vi "SBML Events Handler.vi"(0 "Sim Data w/ time":dbl[][](array[numeric]), 1 "Math Op":string[](array[string]), 2 "Math Val":string[](array[string]), 3 "Var Idx":i32[](array[numeric]), 4 "Idx of Time":i32, 5 "Assign Val":string[][](array[string]), 6 "Delay":dbl[](array[numeric]), 7 "Assign Var Idx":i32[][](array[numeric]), 8 "Flag":i32[](array[numeric]), 9 "Priority":dbl[](array[numeric]), 10 "Delay Val Tot":dbl[](array[numeric]), 11 "Delay Val":dbl) -> (16 "Output Data":dbl[][](array[numeric]), 18 "Flag Out":i32[](array[numeric]), 19 "Delay Val Tot Out":dbl[](array[numeric]))   [LabVIEW 2014]
uses:
  Stop ODE.vi
panel:
  out "Event Idx":i32
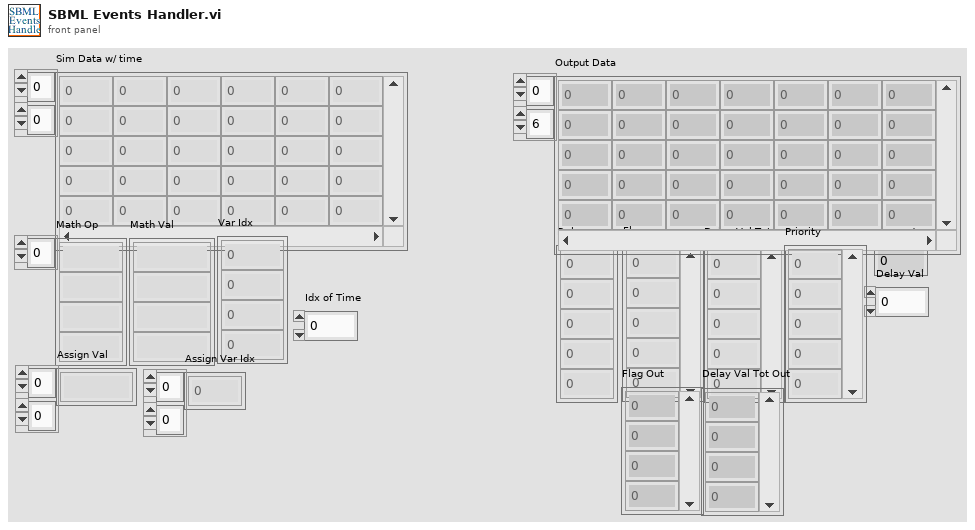
[diagram p1: front panel]
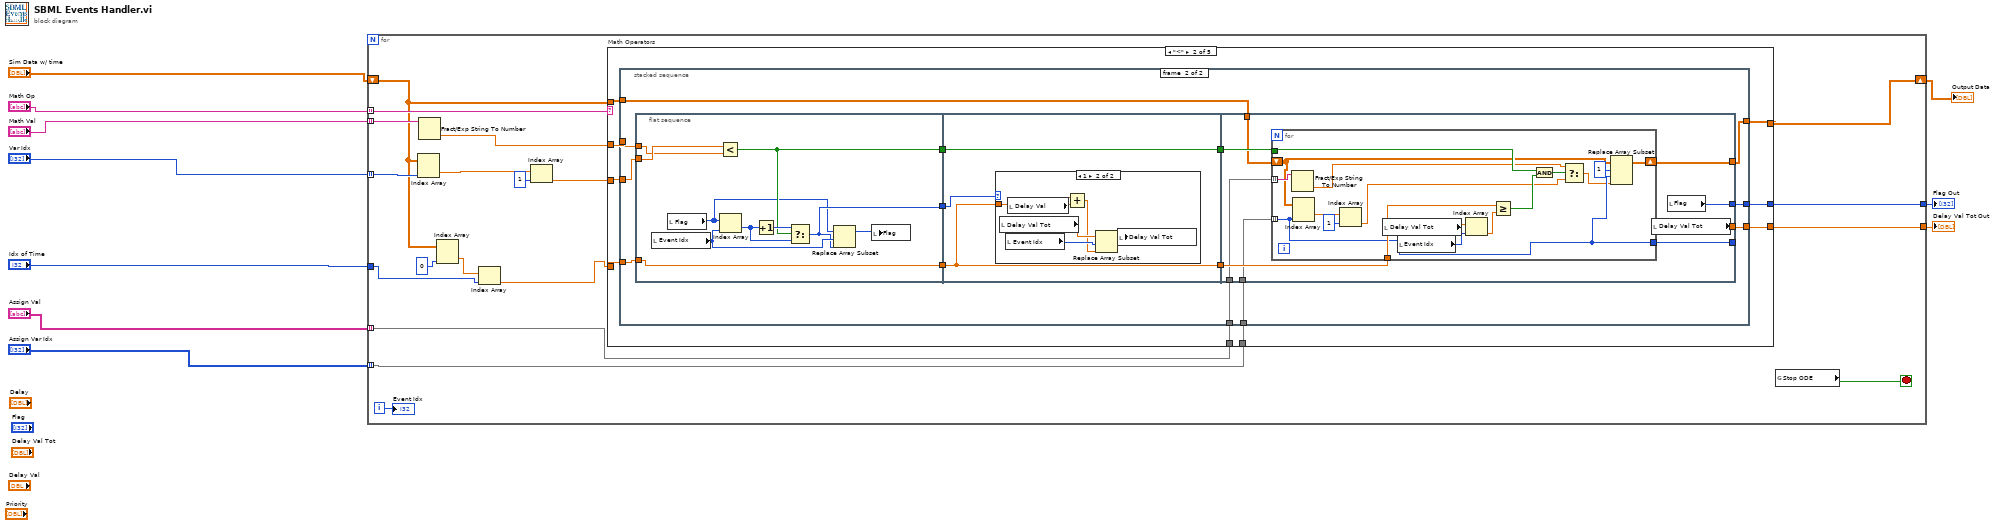
[diagram p0: block diagram]
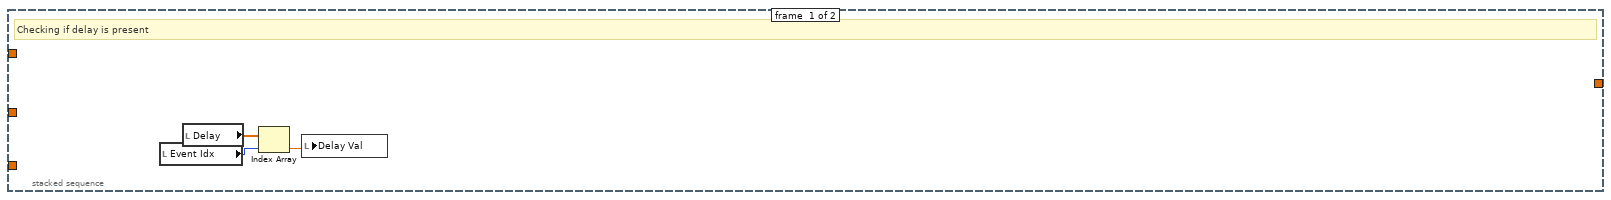
[diagram p3: hidden frame]
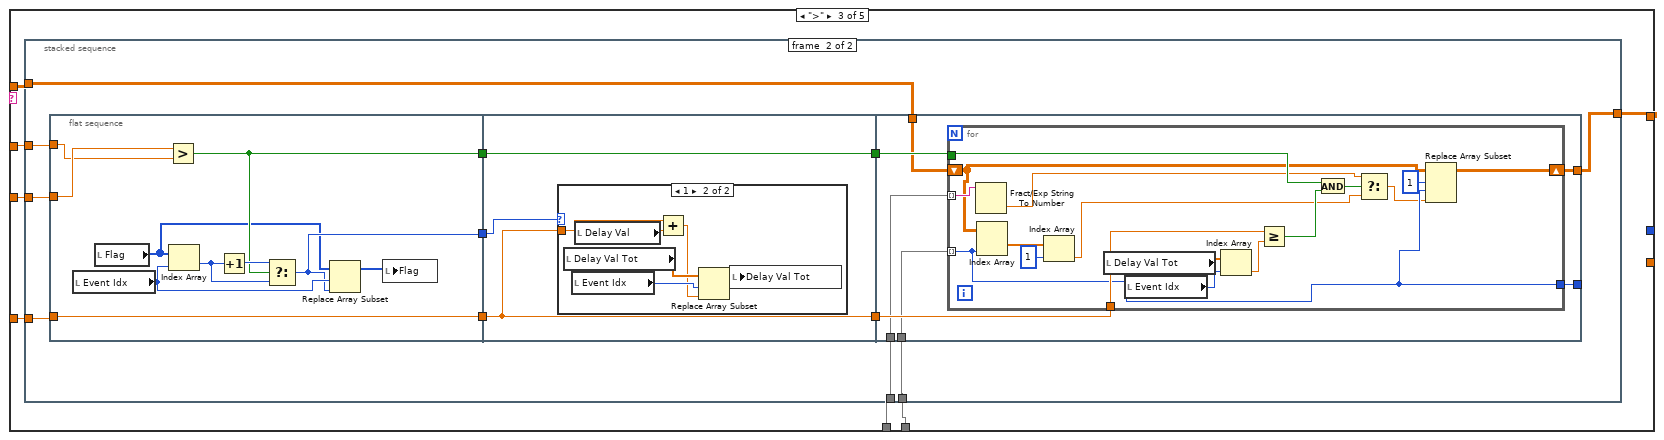
[diagram p5: hidden frame]
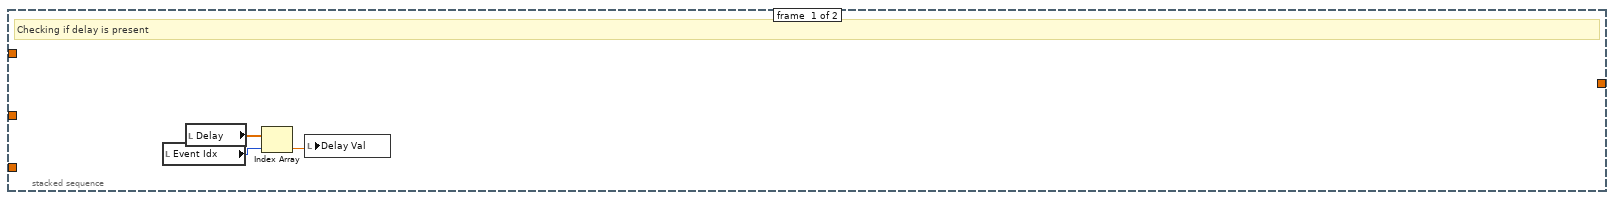
[diagram p6: hidden frame]
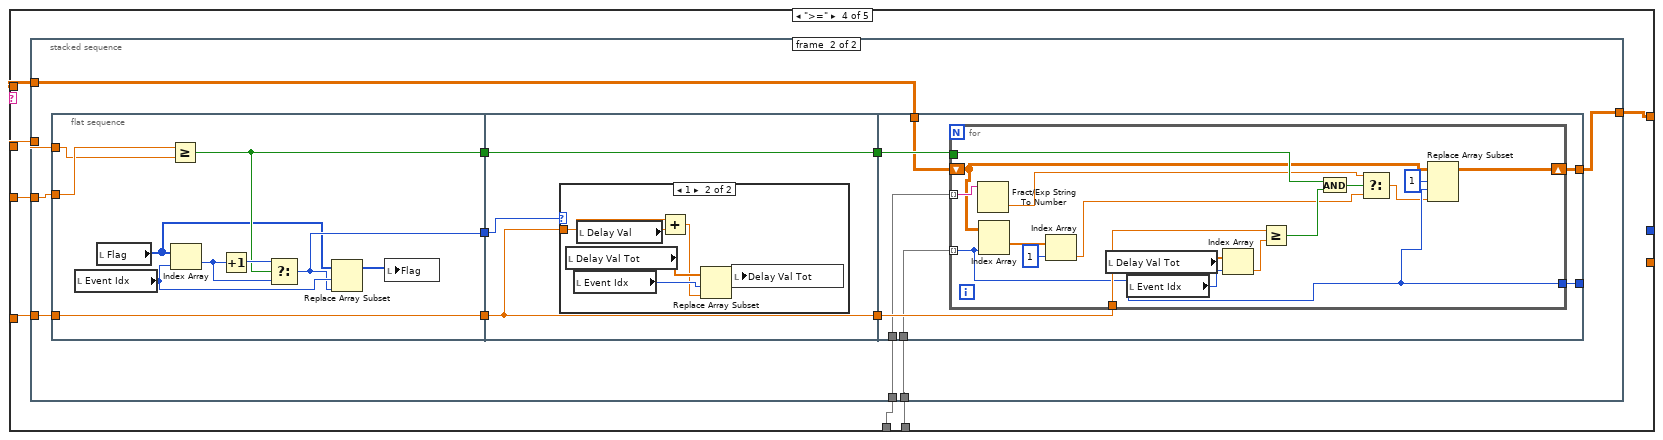
[diagram p8: hidden frame]
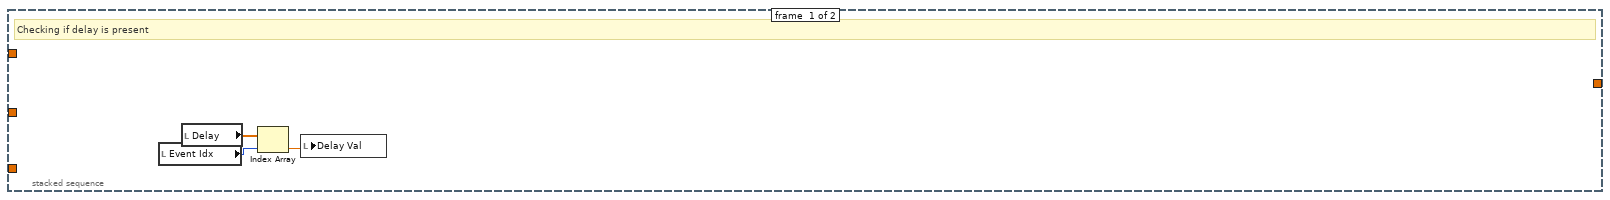
[diagram p9: hidden frame]
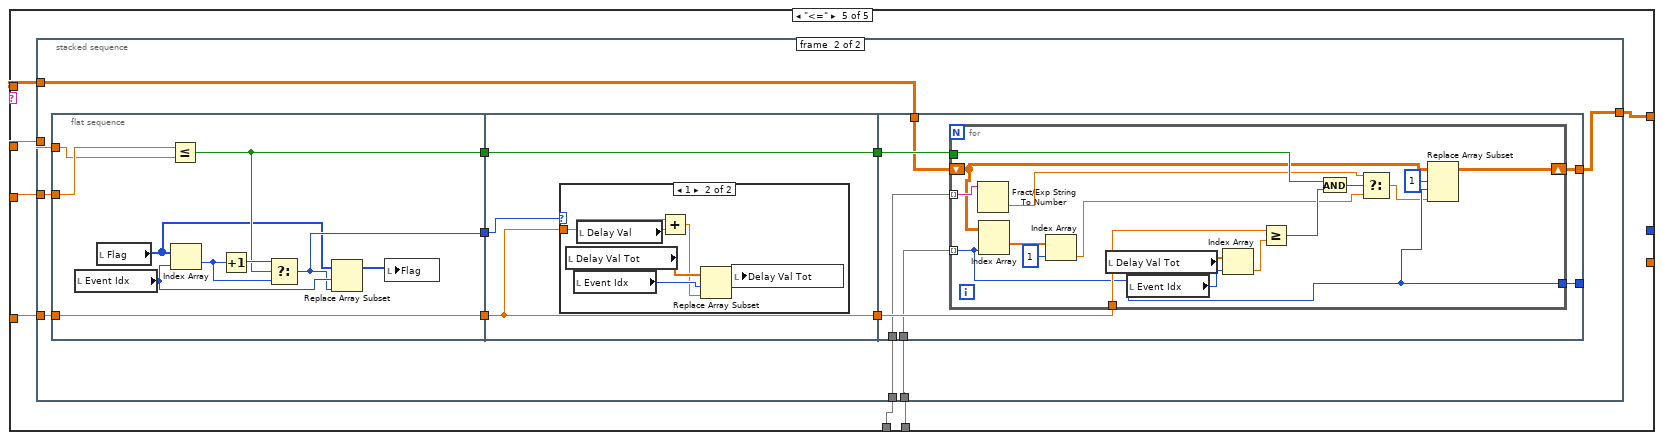
[diagram p11: hidden frame]
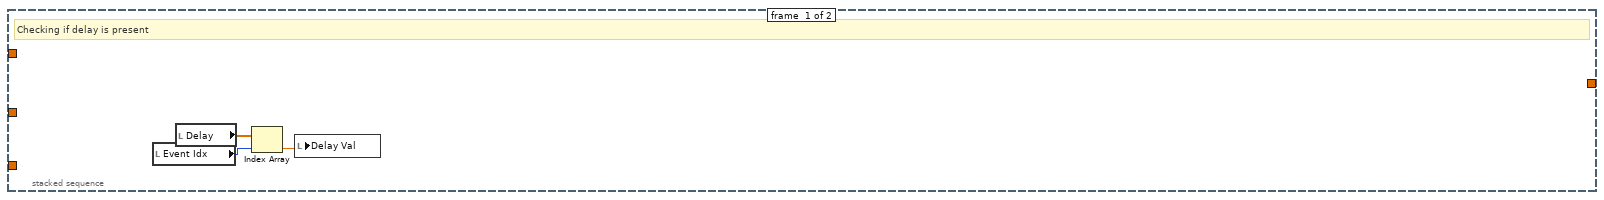
[diagram p12: hidden frame]
diagram:
  n1 = for {
    tunnel: "Math Op" -> [w29] mode=indexing
    tunnel: "Math Val" -> [w28] mode=indexing
    tunnel: "Var Idx" -> [w27] mode=indexing
    tunnel: "Assign Val" -> [w23] mode=indexing
    tunnel: "Assign Var Idx" -> [w26] mode=indexing
    shift-right: [w21] -> w10
    shift-left: "Sim Data w/ time" -> [w15]
    tunnel: "Idx of Time" -> [w13]
    tunnel: [w12] -> w2
    tunnel: [w11] -> w1
    i -> [w24]
    stop <- w25 stop-if-true
    n2 = Index Array(array=w15, index (col)=w27) -> (element=w19:dbl[])  [unwired: 1 in]
    n3 = Fract/Exp String To Number(string=w28) -> (number=w22:dbl)  [unwired: 3 in, 1 out]
    n4 = Index Array(array=w15, index (col)=0 ("disabled index (col)")) -> (element=w17:dbl[])  [unwired: 1 in]
    n5 = Index Array(array=w17, index=w13) -> (element=w14:dbl)
    n6 = Index Array(array=w19, index=1) -> (element=w18:dbl)
    n7 = case "Math Operators" shown="\"<\"" w29 {
      tunnel: w22 -> [_ w37 w106 w171 w236]
      tunnel: [_ w36 w105 w170 w235] -> w21
      tunnel: w15 -> [_ w38 w107 w172 w237]
      tunnel: w23 -> [_ w35 w104 w169 w234]
      tunnel: w26 -> [_ w34 w103 w168 w233]
      tunnel: w18 -> [_ w33 w102 w166 w232]
      tunnel: w14 -> [_ w32 w101 w167 w231]
      tunnel: [_ w31 _ _ _] -> w12
      tunnel: [_ w30 _ _ _] -> w11
      frame "False", Default {
      }
      frame "<" {
        n8 = stacked-sequence {
          tunnel: w37 -> [_ w55]
          tunnel: w38 -> [_ w47]
          tunnel: [_ w46] -> w36
          tunnel: w35 -> [_ w49]
          tunnel: w34 -> [_ w48]
          tunnel: w33 -> [_ w45]
          tunnel: w32 -> [_ w44]
          tunnel: [_ w43] -> w31
          tunnel: [_ w42] -> w30
          frame #0 {
            # "Checking if delay is present"
            n9 = local read "Event Idx"() -> (w40:i32)
            n10 = local read "Delay"() -> (w41:dbl[])
            n11 = Index Array(array=w41, index=w40) -> (element=w39:dbl)
            n12 = local write "Delay Val"(w39) -> ()
          }
          frame #1 {
            n13 = flat-sequence {
              tunnel: w45 -> [w65]
              tunnel: w55 -> [w64]
              tunnel: [w59] -> w54
              tunnel: [w58] -> w53
              tunnel: [w56] -> w52
              tunnel: w44 -> [w56]
              tunnel: w54 -> [w67]
              tunnel: w53 -> [w68]
              tunnel: w52 -> [w66]
              tunnel: [w68] -> w51
              tunnel: [w66] -> w50
              tunnel: w51 -> [w83]
              tunnel: w50 -> [w82]
              tunnel: w47 -> [w81]
              tunnel: w48 -> [w80]
              tunnel: w49 -> [w79]
              tunnel: [w78] -> _
              tunnel: [w77] -> w46
              tunnel: [w76] -> w43
              tunnel: [w75] -> w42
              frame #0 {
                n14 = local read "Event Idx"() -> (w62:i32)
                n15 = local read "Flag"() -> (w57:i32[])
                n16 = Less?(x=w65, y=w64) -> (x < y?=w58:bool)
                n17 = Index Array(array=w57, index=w62) -> (element=w61:i32)
                n18 = Increment(x=w61) -> (x+1=w60:i32)
                n19 = Select(t=w60, s=w58, f=w61) -> (s? t:f=w59:i32)
                n20 = Replace Array Subset(array=w57, new element=w59, index=w62) -> (w63:i32[])
                n21 = local write "Flag"(w63) -> ()
              }
              frame #1 {
                n22 = case shown="1" w67 {
                  tunnel: w66 -> [_ w73]
                  frame 0, Default {
                  }
                  frame 1 {
                    n23 = local read "Delay Val Tot"() -> (w72:dbl[])
                    n24 = local read "Event Idx"() -> (w70:i32)
                    n25 = local read "Delay Val"() -> (w74:dbl)
                    n26 = Add(x=w73, y=w74) -> (x+y=w69:dbl)
                    n27 = Replace Array Subset(array=w72, new element=w69, index=w70) -> (w71:dbl[])
                    n28 = local write "Delay Val Tot"(w71) -> ()
                  }
                }
              }
              frame #2 {
                n29 = for {
                  tunnel: w83 -> [w98]
                  tunnel: w82 -> [w97]
                  tunnel: w80 -> [w87] mode=indexing
                  tunnel: w79 -> [w90] mode=indexing
                  tunnel: [w87] -> w78
                  shift-right: [w85] -> w77
                  shift-left: w81 -> [w84]
                  n30 = Fract/Exp String To Number(string=w90) -> (number=w89:dbl)  [unwired: 3 in, 1 out]
                  n31 = Index Array(array=w84, index (col)=w87) -> (element=w92:dbl[])  [unwired: 1 in]
                  n32 = Index Array(array=w92, index=1) -> (element=w91:dbl)
                  n33 = local read "Delay Val Tot"() -> (w96:dbl[])
                  n34 = local read "Event Idx"() -> (w95:i32)
                  n35 = Index Array(array=w96, index=w95) -> (element=w94:dbl)
                  n36 = Greater Or Equal?(x=w97, y=w94) -> (x >= y?=w99:bool)
                  n37 = And(x=w98, y=w99) -> (x .and. y?=w100:bool)
                  n38 = Select(t=w89, s=w100, f=w91) -> (s? t:f=w86:dbl)
                  n39 = Replace Array Subset(array=w84, new element=w86, index (row)=1, index (col)=w87) -> (w85:dbl[][])
                }
                n40 = local read "Delay Val Tot"() -> (w75:dbl[])
                n41 = local read "Flag"() -> (w76:i32[])
              }
            }
          }
        }
      }
      frame ">" {
        n42 = stacked-sequence {
          tunnel: w106 -> [_ w122]
          tunnel: w107 -> [_ w114]
          tunnel: [_ w113] -> w105
          tunnel: w104 -> [_ w116]
          tunnel: w103 -> [_ w115]
          tunnel: w102 -> [_ w112]
          tunnel: w101 -> [_ w111]
          frame #0 {
            # "Checking if delay is present"
            n43 = local read "Event Idx"() -> (w109:i32)
            n44 = local read "Delay"() -> (w110:dbl[])
            n45 = Index Array(array=w110, index=w109) -> (element=w108:dbl)
            n46 = local write "Delay Val"(w108) -> ()
          }
          frame #1 {
            n47 = flat-sequence {
              tunnel: w112 -> [w132]
              tunnel: w122 -> [w131]
              tunnel: w111 -> [w130]
              tunnel: [w125] -> w121
              tunnel: [w124] -> w120
              tunnel: [w130] -> w119
              tunnel: w121 -> [w134]
              tunnel: w120 -> [w135]
              tunnel: w119 -> [w133]
              tunnel: [w135] -> w118
              tunnel: [w133] -> w117
              tunnel: w118 -> [w148]
              tunnel: w117 -> [w147]
              tunnel: w114 -> [w146]
              tunnel: w115 -> [w145]
              tunnel: w116 -> [w144]
              tunnel: [w143] -> _
              tunnel: [w142] -> w113
              frame #0 {
                n48 = local read "Event Idx"() -> (w128:i32)
                n49 = local read "Flag"() -> (w123:i32[])
                n50 = Greater?(x=w132, y=w131) -> (0:w124:bool)
                n51 = Index Array(array=w123, index=w128) -> (element=w127:i32)
                n52 = Increment(x=w127) -> (x+1=w126:i32)
                n53 = Select(t=w126, s=w124, f=w127) -> (s? t:f=w125:i32)
                n54 = Replace Array Subset(array=w123, new element=w125, index=w128) -> (w129:i32[])
                n55 = local write "Flag"(w129) -> ()
              }
              frame #1 {
                n56 = case shown="1" w134 {
                  tunnel: w133 -> [_ w140]
                  frame 0, Default {
                  }
                  frame 1 {
                    n57 = local read "Delay Val Tot"() -> (w139:dbl[])
                    n58 = local read "Event Idx"() -> (w137:i32)
                    n59 = local read "Delay Val"() -> (w141:dbl)
                    n60 = Add(x=w140, y=w141) -> (x+y=w136:dbl)
                    n61 = Replace Array Subset(array=w139, new element=w136, index=w137) -> (w138:dbl[])
                    n62 = local write "Delay Val Tot"(w138) -> ()
                  }
                }
              }
              frame #2 {
                n63 = for {
                  tunnel: w148 -> [w163]
                  tunnel: w147 -> [w162]
                  tunnel: w145 -> [w152] mode=indexing
                  tunnel: w144 -> [w155] mode=indexing
                  tunnel: [w152] -> w143
                  shift-right: [w150] -> w142
                  shift-left: w146 -> [w149]
                  n64 = Fract/Exp String To Number(string=w155) -> (number=w154:dbl)  [unwired: 3 in, 1 out]
                  n65 = Index Array(array=w149, index (col)=w152) -> (element=w157:dbl[])  [unwired: 1 in]
                  n66 = Index Array(array=w157, index=1) -> (element=w156:dbl)
                  n67 = local read "Delay Val Tot"() -> (w161:dbl[])
                  n68 = local read "Event Idx"() -> (w160:i32)
                  n69 = Index Array(array=w161, index=w160) -> (element=w159:dbl)
                  n70 = Greater Or Equal?(x=w162, y=w159) -> (x >= y?=w164:bool)
                  n71 = And(x=w163, y=w164) -> (x .and. y?=w165:bool)
                  n72 = Select(t=w154, s=w165, f=w156) -> (s? t:f=w151:dbl)
                  n73 = Replace Array Subset(array=w149, new element=w151, index (row)=1, index (col)=w152) -> (w150:dbl[][])
                }
              }
            }
          }
        }
      }
      frame ">=" {
        n74 = stacked-sequence {
          tunnel: w171 -> [_ w187]
          tunnel: w172 -> [_ w179]
          tunnel: [_ w178] -> w170
          tunnel: w169 -> [_ w181]
          tunnel: w168 -> [_ w180]
          tunnel: w167 -> [_ w177]
          tunnel: w166 -> [_ w176]
          frame #0 {
            # "Checking if delay is present"
            n75 = local read "Event Idx"() -> (w174:i32)
            n76 = local read "Delay"() -> (w175:dbl[])
            n77 = Index Array(array=w175, index=w174) -> (element=w173:dbl)
            n78 = local write "Delay Val"(w173) -> ()
          }
          frame #1 {
            n79 = flat-sequence {
              tunnel: w176 -> [w197]
              tunnel: w187 -> [w196]
              tunnel: w177 -> [w195]
              tunnel: [w190] -> w186
              tunnel: [w189] -> w185
              tunnel: [w195] -> w184
              tunnel: w186 -> [w199]
              tunnel: w185 -> [w200]
              tunnel: w184 -> [w198]
              tunnel: [w200] -> w183
              tunnel: [w198] -> w182
              tunnel: w183 -> [w213]
              tunnel: w182 -> [w212]
              tunnel: w179 -> [w211]
              tunnel: w180 -> [w210]
              tunnel: w181 -> [w209]
              tunnel: [w208] -> _
              tunnel: [w207] -> w178
              frame #0 {
                n80 = local read "Event Idx"() -> (w193:i32)
                n81 = local read "Flag"() -> (w188:i32[])
                n82 = Greater Or Equal?(x=w197, y=w196) -> (x >= y?=w189:bool)
                n83 = Index Array(array=w188, index=w193) -> (element=w192:i32)
                n84 = Increment(x=w192) -> (x+1=w191:i32)
                n85 = Select(t=w191, s=w189, f=w192) -> (s? t:f=w190:i32)
                n86 = Replace Array Subset(array=w188, new element=w190, index=w193) -> (w194:i32[])
                n87 = local write "Flag"(w194) -> ()
              }
              frame #1 {
                n88 = case shown="1" w199 {
                  tunnel: w198 -> [_ w205]
                  frame 0, Default {
                  }
                  frame 1 {
                    n89 = local read "Delay Val Tot"() -> (w204:dbl[])
                    n90 = local read "Event Idx"() -> (w202:i32)
                    n91 = local read "Delay Val"() -> (w206:dbl)
                    n92 = Add(x=w205, y=w206) -> (x+y=w201:dbl)
                    n93 = Replace Array Subset(array=w204, new element=w201, index=w202) -> (w203:dbl[])
                    n94 = local write "Delay Val Tot"(w203) -> ()
                  }
                }
              }
              frame #2 {
                n95 = for {
                  tunnel: w213 -> [w228]
                  tunnel: w212 -> [w227]
                  tunnel: w210 -> [w217] mode=indexing
                  tunnel: w209 -> [w220] mode=indexing
                  tunnel: [w217] -> w208
                  shift-right: [w215] -> w207
                  shift-left: w211 -> [w214]
                  n96 = Fract/Exp String To Number(string=w220) -> (number=w219:dbl)  [unwired: 3 in, 1 out]
                  n97 = Index Array(array=w214, index (col)=w217) -> (element=w222:dbl[])  [unwired: 1 in]
                  n98 = Index Array(array=w222, index=1) -> (element=w221:dbl)
                  n99 = local read "Delay Val Tot"() -> (w226:dbl[])
                  n100 = local read "Event Idx"() -> (w225:i32)
                  n101 = Index Array(array=w226, index=w225) -> (element=w224:dbl)
                  n102 = Greater Or Equal?(x=w227, y=w224) -> (x >= y?=w229:bool)
                  n103 = And(x=w228, y=w229) -> (x .and. y?=w230:bool)
                  n104 = Select(t=w219, s=w230, f=w221) -> (s? t:f=w216:dbl)
                  n105 = Replace Array Subset(array=w214, new element=w216, index (row)=1, index (col)=w217) -> (w215:dbl[][])
                }
              }
            }
          }
        }
      }
      frame "<=" {
        n106 = stacked-sequence {
          tunnel: w236 -> [_ w252]
          tunnel: w237 -> [_ w244]
          tunnel: [_ w243] -> w235
          tunnel: w234 -> [_ w246]
          tunnel: w233 -> [_ w245]
          tunnel: w232 -> [_ w242]
          tunnel: w231 -> [_ w241]
          frame #0 {
            # "Checking if delay is present"
            n107 = local read "Event Idx"() -> (w239:i32)
            n108 = local read "Delay"() -> (w240:dbl[])
            n109 = Index Array(array=w240, index=w239) -> (element=w238:dbl)
            n110 = local write "Delay Val"(w238) -> ()
          }
          frame #1 {
            n111 = flat-sequence {
              tunnel: w242 -> [w262]
              tunnel: w252 -> [w261]
              tunnel: w241 -> [w260]
              tunnel: [w255] -> w251
              tunnel: [w254] -> w250
              tunnel: [w260] -> w249
              tunnel: w251 -> [w264]
              tunnel: w250 -> [w265]
              tunnel: w249 -> [w263]
              tunnel: [w265] -> w248
              tunnel: [w263] -> w247
              tunnel: w248 -> [w278]
              tunnel: w247 -> [w277]
              tunnel: w244 -> [w276]
              tunnel: w245 -> [w275]
              tunnel: w246 -> [w274]
              tunnel: [w273] -> _
              tunnel: [w272] -> w243
              frame #0 {
                n112 = local read "Event Idx"() -> (w258:i32)
                n113 = local read "Flag"() -> (w253:i32[])
                n114 = Less Or Equal?(x=w262, y=w261) -> (x <= y?=w254:bool)
                n115 = Index Array(array=w253, index=w258) -> (element=w257:i32)
                n116 = Increment(x=w257) -> (x+1=w256:i32)
                n117 = Select(t=w256, s=w254, f=w257) -> (s? t:f=w255:i32)
                n118 = Replace Array Subset(array=w253, new element=w255, index=w258) -> (w259:i32[])
                n119 = local write "Flag"(w259) -> ()
              }
              frame #1 {
                n120 = case shown="1" w264 {
                  tunnel: w263 -> [_ w270]
                  frame 0, Default {
                  }
                  frame 1 {
                    n121 = local read "Delay Val Tot"() -> (w269:dbl[])
                    n122 = local read "Event Idx"() -> (w267:i32)
                    n123 = local read "Delay Val"() -> (w271:dbl)
                    n124 = Add(x=w270, y=w271) -> (x+y=w266:dbl)
                    n125 = Replace Array Subset(array=w269, new element=w266, index=w267) -> (w268:dbl[])
                    n126 = local write "Delay Val Tot"(w268) -> ()
                  }
                }
              }
              frame #2 {
                n127 = for {
                  tunnel: w278 -> [w293]
                  tunnel: w277 -> [w292]
                  tunnel: w275 -> [w282] mode=indexing
                  tunnel: w274 -> [w285] mode=indexing
                  tunnel: [w282] -> w273
                  shift-right: [w280] -> w272
                  shift-left: w276 -> [w279]
                  n128 = Fract/Exp String To Number(string=w285) -> (number=w284:dbl)  [unwired: 3 in, 1 out]
                  n129 = Index Array(array=w279, index (col)=w282) -> (element=w287:dbl[])  [unwired: 1 in]
                  n130 = Index Array(array=w287, index=1) -> (element=w286:dbl)
                  n131 = local read "Delay Val Tot"() -> (w291:dbl[])
                  n132 = local read "Event Idx"() -> (w290:i32)
                  n133 = Index Array(array=w291, index=w290) -> (element=w289:dbl)
                  n134 = Greater Or Equal?(x=w292, y=w289) -> (x >= y?=w294:bool)
                  n135 = And(x=w293, y=w294) -> (x .and. y?=w295:bool)
                  n136 = Select(t=w284, s=w295, f=w286) -> (s? t:f=w281:dbl)
                  n137 = Replace Array Subset(array=w279, new element=w281, index (row)=1, index (col)=w282) -> (w280:dbl[][])
                }
              }
            }
          }
        }
      }
    }
    n138 = global read "Stop ODE.vi" "Stop ODE"() -> (w25:bool)
    "Event Idx" <- w24
  }
  "Output Data" <- w10
  "Flag Out" <- w2
  "Delay Val Tot Out" <- w1
